vi "Solver2.vi"(11 "Previous Guess Result":string) -> (3 "New Guess":string)   [LabVIEW 2022 SP3]
uses:
  <vilib>/numeric/sub_Random U32.vi
  <vilib>/numeric/Random Number (Range) I64.vi
  Libraries/Wordle Engine/Wordle Engine.lvlib
panel:
  out "Valid Guesses (array) 2":string[](array[string])
  out "starting guess":string
  out "Database Size":i32
  out "index":u64
  out "Valid Guesses (array)":string[](array[string])
  # "Note: Do not change the connector pane of this VI."
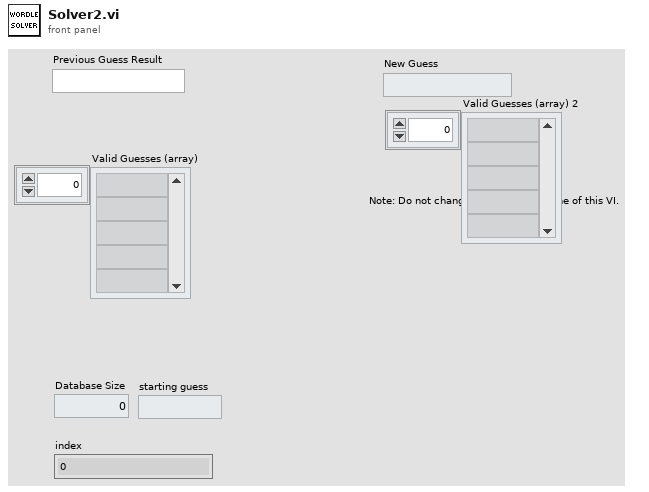
[diagram p1: front panel]
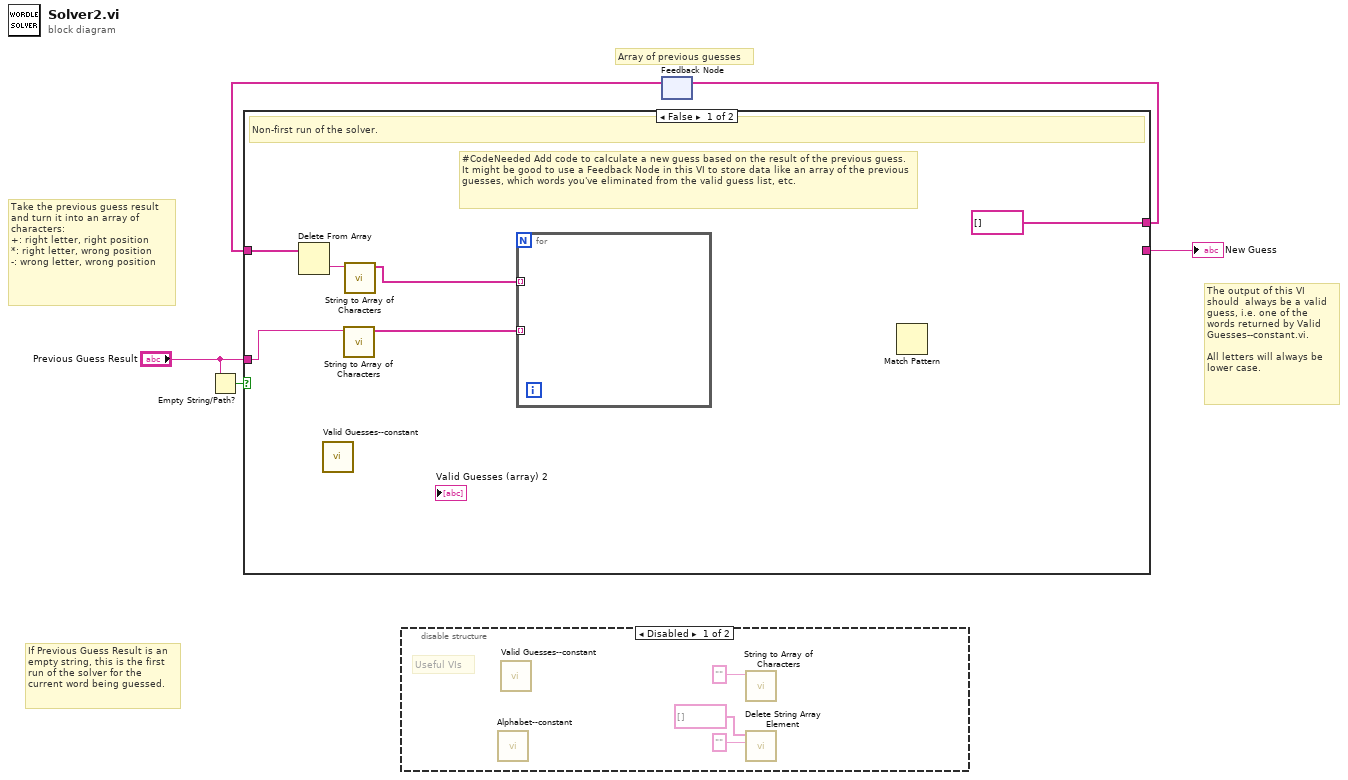
[diagram p0: block diagram]
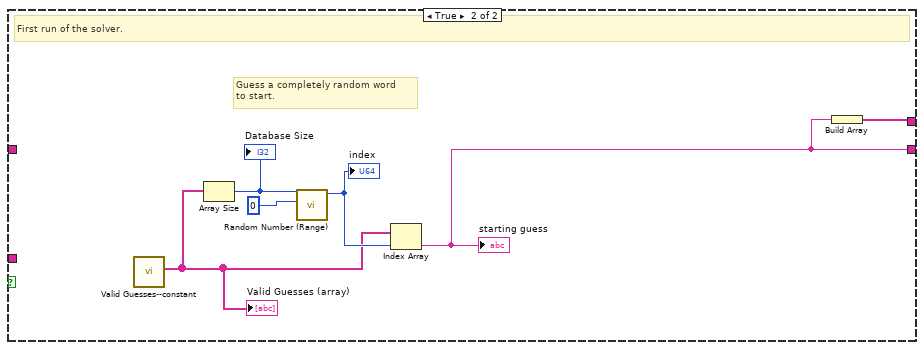
[diagram p2: hidden frame]
diagram:
  # "Array of previous guesses"
  # "Take the previous guess result and turn it into an array of characters:\n+: right letter, right position\n*: right letter, wrong position\n-: wrong letter, wrong position"
  # "The output of this VI should  always be a valid guess, i.e. one of the words returned by Valid Guesses--constant.vi.\n\nAll letters will always be lower case."
  # "If Previous Guess Result is an empty string, this is the first run of the solver for the current word being guessed."
  n1 = Empty String/Path?(string/path="Previous Guess Result") -> (empty?=w4:bool)
  n2 = disable-structure shown="Disabled" {
    frame Disabled {
      # "Useful VIs"
      n3 = call "Alphabet--constant.vi"() -> ()  [unwired: 10 in, 2 out]
      n4 = call "Valid Guesses--constant.vi"() -> ()  [unwired: 10 in, 2 out]
      n5 = call "String to Array of Characters.vi"("String"="") -> ()  [unwired: 10 in, 1 out]
      n6 = call "Delete String Array Element.vi"("Element to Delete"="", "Array in"=string[] []) -> ()  [unwired: 8 in, 2 out]
    }
    frame Enabled {
    }
  }
  n7 = feedback #1() -> (w2:string[])  [unwired: 1 in]
  n8 = case shown="False" w4 {
    tunnel: [_ w15] -> w3
    tunnel: "Previous Guess Result" -> [w13 _]
    tunnel: w2 -> [w11 _]
    tunnel: [string[] [] ("String") w16] -> w1
    frame False {
      # "#CodeNeeded Add code to calculate a new guess based on the result of the previous guess. It might be good to use a Feedback Node in this VI to store data like an array of the previous guesses, which words you've eliminated from the valid guess list, etc."
      # "Non-first run of the solver."
      n9 = Delete From Array(array=w11) -> (deleted portion=w10:string)  [unwired: 2 in, 1 out]
      n10 = call "Valid Guesses--constant.vi"() -> ()  [unwired: 10 in, 2 out]
      n11 = call "String to Array of Characters.vi"("String"=w13) -> ("Array of Characters"=w12:string[])  [unwired: 10 in]
      n12 = call "String to Array of Characters.vi"("String"=w10) -> ("Array of Characters"=w9:string[])  [unwired: 10 in]
      n13 = for {
        tunnel: w12 -> [_] mode=indexing
        tunnel: w9 -> [_] mode=indexing
      }
      n14 = Match Pattern() -> ()  [unwired: 3 in, 4 out]
    }
    frame True {
      # "Guess a completely random word \nto start."
      # "First run of the solver."
      n15 = call "Valid Guesses--constant.vi"() -> ("Valid Guesses (array)"=w17:string[])  [unwired: 10 in, 1 out]
      "Valid Guesses (array)" <- w17
      n16 = Array Size(array=w17) -> (size(s)=w20:i32)
      "Database Size" <- w20
      n17 = call-poly <vilib>:"Random Number (Range).vi"("lower bound (-100)"=i64 0, "upper bound (100)"=w20) -> ("number"=w18:i64)  [unwired: 9 in]
      "index" <- w18
      n18 = Index Array(array=w17, index=w18) -> (element=w15:string)
      "starting guess" <- w15
      n19 = Build Array(w15) -> (w16:string[])
    }
  }
  "New Guess" <- w3
  n20 = feedback-in #1(w1) -> ()
